vi "Get Generation Registers.vi"(2 "gen":refnum<class "niUSRP Tx DSP v2 FPGA.lvclass">) -> (4 "gen registers":T1)   [LabVIEW 2025, in "niUSRP Tx DSP v2 FPGA.lvclass"]
uses:
  niUSRP Tx DSP v2 FPGA.lvclass
  <instrlib>/_niInstr/Instruction Framework/v1/FPGA/Interfaces/Address Space Collection/Address Space Collection.lvclass
  niUSRP Tx DSP v2 FPGA.lvclass/niUSRP Tx DSP v2 FPGA.ctl
  <instrlib>/_niInstr/Basic Elements/v1/FPGA/niInstr Basic Elements v1 FPGA.lvlib
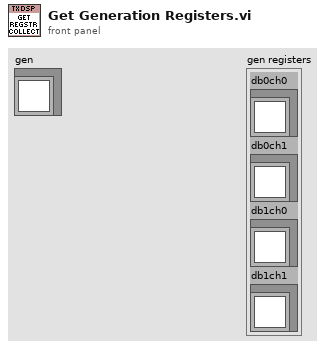
[diagram p1: front panel]
types:
  T1 = cluster{"db0ch0":refnum<class "Address Space Collection.lvclass">, "db0ch1":refnum<class "Address Space Collection.lvclass">, "db1ch0":refnum<class "Address Space Collection.lvclass">, "db1ch1":refnum<class "Address Space Collection.lvclass">}
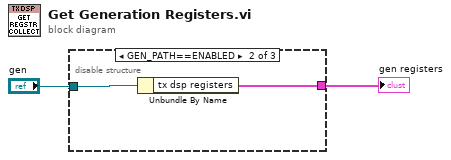
[diagram p0: block diagram]
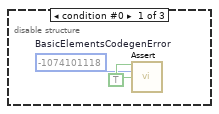
[diagram p2: hidden frame]
diagram:
  n1 = disable-structure shown="GEN_PATH==ENABLED" {
    disable-tunnel: "gen" -> [_ w6 _]
    disable-tunnel: [_ w5 _] -> w1
    frame condition #0 {
      w4 = TRUE ("assert")
      w3 = -1074101118  # BasicElementsCodegenError
      n2 = call <instrlib>:"Assert.vi"("assert"=w4, "error code"=w3, "enable show error"=w4) -> ()  [unwired: 13 in]
    }
    frame condition #1 (active) {
      n3 = Unbundle By Name(w6) -> ("tx dsp registers"=w5:T1)
    }
    frame condition #2 {
    }
  }
  "gen registers" <- w1
